vi "Drag-Drop Change.vi"(7 "Action":T1, 10 "Mouse Interaction Tag":string, 11 "UI Data In":refnum<class "Settings UI.lvclass">) -> (3 "UI Data Out":refnum<class "Settings UI.lvclass">)   [LabVIEW 2020, in "Output Sequencer.lvlib" / "Settings UI.lvclass"]
uses:
  Settings UI.lvclass
  Types/Settings UI Action.ctl
  Settings UI.lvclass/Settings UI.ctl
  Types/Drag-Drop State.ctl
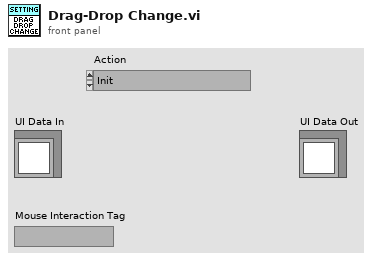
[diagram p1: front panel]
types:
  T1 = typedef "Output Sequencer.lvlib/Settings UI.lvclass/Settings UI Action.ctl" = enum16{"Init", "Timeout", "Tree Change", "Tree Mouse Down/Up", "Value Change", "Expand All", "Show Overview", "Collapse All", "Insert Above", "Insert Below", "Remove Step", "Move Up", "Move Down", "Drag Starting", "Drag Over", "Drop", "Drag Ended", "Import"}
  T2 = typedef "Output Sequencer.lvlib/Settings UI.lvclass/Drag-Drop State.ctl" = cluster{"Step Number":i32, "Current Index":i32, "Dropped?":bool, "Previous Open State":bool[]}
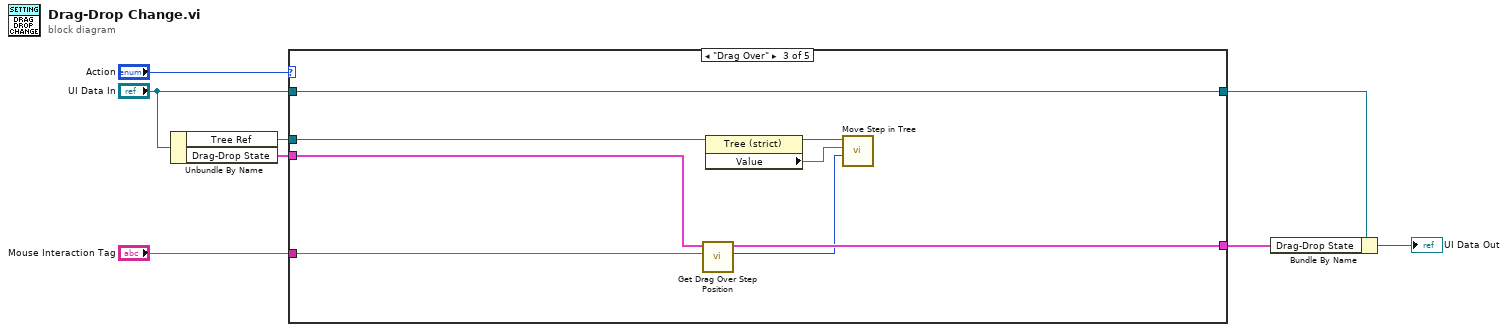
[diagram p0: block diagram]
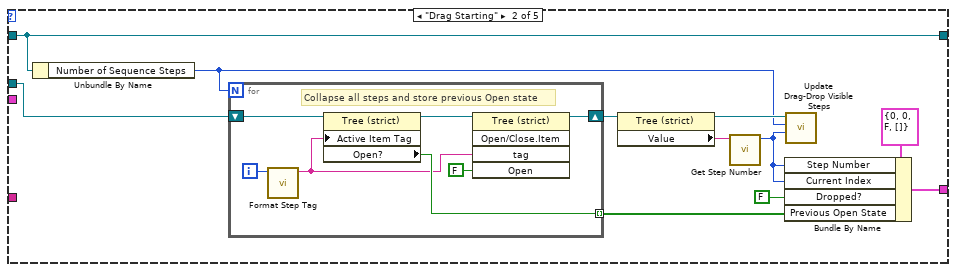
[diagram p3: hidden frame]
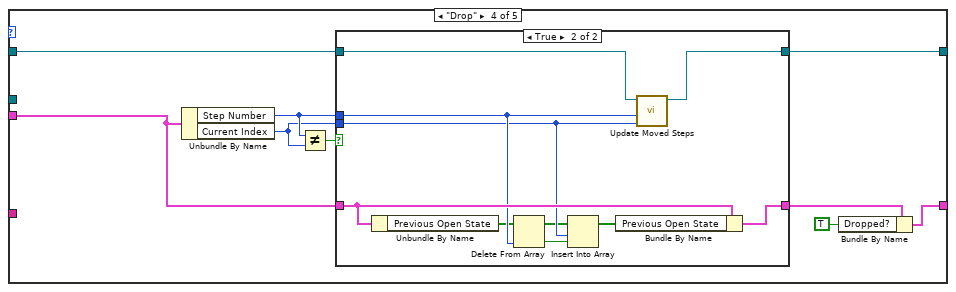
[diagram p4: hidden frame]
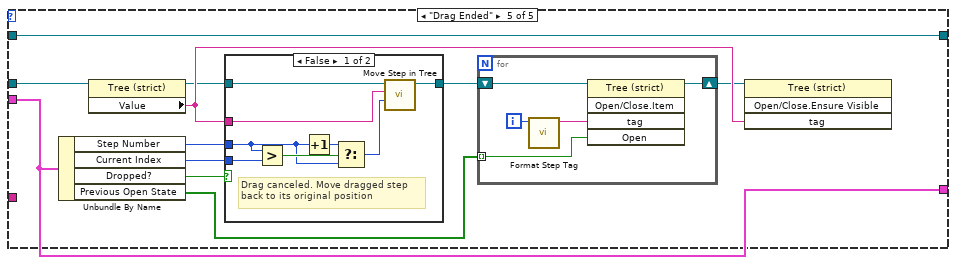
[diagram p6: hidden frame]
diagram:
  n1 = Unbundle By Name("UI Data In") -> ("Tree Ref"=w5:refnum<vi>, "Drag-Drop State"=w4:T2)
  n2 = case shown="\"Drag Over\"" "Action" {
    tunnel: w4 -> [w10 _ w35 w39 w67]
    tunnel: [w10 w19 w32 w37 w67] -> w1
    tunnel: "Mouse Interaction Tag" -> [_ _ w36 _ _]
    tunnel: "UI Data In" -> [w9 w18 w34 w44 w64]
    tunnel: [w9 w18 w34 w40 w64] -> w3
    tunnel: w5 -> [_ w11 w31 _ w58]
    frame Default {
    }
    frame "Drag Starting" {
      n3 = Unbundle By Name(w18) -> ("Number of Sequence Steps"=w13:i32)
      n4 = for {
        N: w13 -> [_]
        shift-right: [w27] -> w15
        shift-left: w11 -> [w26]
        tunnel: [w24] -> w17 mode=indexing
        i -> [w22]
        # "Collapse all steps and store previous Open state"
        n5 = call "Format Step Tag.vi"("Step Number"=w22) -> ("Tag"=w23:string)  [unwired: 10 in]
        n6 = property class="Tree (strict)"(reference=w26, "Active Item Tag"=w23) -> (reference out=w25:refnum<vi>, "Open?"=w24:bool)  [unwired: 1 in, 1 out]
        n7 = invoke class="Tree (strict)" method="Open/Close.Item"(reference=w25, "tag"=w23, "Open"=FALSE ("Open?")) -> (reference out=w27:refnum<vi>)  [unwired: 2 in, 4 out]
      }
      n8 = property class="Tree (strict)"(reference=w15) -> (reference out=w14:refnum<vi>, "Value"=w21:string)  [unwired: 1 in, 1 out]
      n9 = call "Get Step Number.vi"("Tree Tag"=w21) -> ("Step Number"=w12:i32)  [unwired: 8 in, 2 out]
      n10 = Bundle By Name(cluster=T2 {"Step Number"=0, "Current Index"=0, "Dropped?"=FALSE, "Previous Open State"=[]} ("Drag-Drop State in"), "Step Number"=w12, "Current Index"=w12, "Dropped?"=FALSE, "Previous Open State"=w17) -> (w19:T2)
      n11 = call "Update Drag-Drop Visible Steps.vi"("Step Number"=w12, "Number of Sequence Steps"=w13, "TreeControl in"=w14) -> ()  [unwired: 9 in]
    }
    frame "Drag Over" {
      n12 = call "Get Drag Over Step Position.vi"("Mouse Interaction Tag"=w36, "Drag-Drop State in"=w35) -> ("New Position"=w29:i32, "Drag-Drop State out"=w32:T2)  [unwired: 8 in]
      n13 = property class="Tree (strict)"(reference=w31) -> (reference out=w33:refnum<vi>, "Value"=w30:string)  [unwired: 1 in, 1 out]
      n14 = call "Move Step in Tree.vi"("New Position"=w29, "Step Tag"=w30, "TreeControl in"=w33) -> ()  [unwired: 8 in, 1 out]
    }
    frame "Drop" {
      n15 = Unbundle By Name(w39) -> ("Step Number"=w43:i32, "Current Index"=w42:i32)
      n16 = Not Equal?(x=w43, y=w42) -> (x != y?=w41:bool)
      n17 = case shown="True" w41 {
        tunnel: w44 -> [w47 w49]
        tunnel: w42 -> [_ w55]
        tunnel: w43 -> [_ w56]
        tunnel: [w47 w48] -> w40
        tunnel: w39 -> [w46 w57]
        tunnel: [w46 w54] -> w38
        frame False {
        }
        frame True {
          n18 = Unbundle By Name(w57) -> ("Previous Open State"=w53:bool[])
          n19 = Delete From Array(array=w53, index=w56) -> (deleted portion=w51:bool, array with subset deleted=w52:bool[])  [unwired: 1 in]
          n20 = Insert Into Array(array=w52, index=w55, new element=w51) -> (w50:bool[])
          n21 = Bundle By Name(cluster=w57, "Previous Open State"=w50) -> (w54:T2)
          n22 = call "Update Moved Steps.vi"("New Step Number"=w55, "Previous Step Number"=w56, "UI Data In"=w49) -> ("UI Data Out"=w48:refnum<class "Settings UI.lvclass">)  [unwired: 8 in]
        }
      }
      n23 = Bundle By Name(cluster=w38, "Dropped?"=TRUE) -> (w37:T2)
    }
    frame "Drag Ended" {
      n24 = Unbundle By Name(w67) -> ("Step Number"=w65:i32, "Current Index"=w66:i32, "Dropped?"=w60:bool, "Previous Open State"=w59:bool[])
      n25 = property class="Tree (strict)"(reference=w58) -> (reference out=w61:refnum<vi>, "Value"=w68:string)  [unwired: 1 in, 1 out]
      n26 = case shown="False" w60 {
        tunnel: w61 -> [w75 w82]
        tunnel: [w74 w82] -> w62
        tunnel: w68 -> [w77 _]
        tunnel: w66 -> [w79 _]
        tunnel: w65 -> [w78 _]
        frame False {
          # "Drag canceled. Move dragged step\nback to its original position"
          n27 = Greater?(x=w78, y=w79) -> (0:w81:bool)
          n28 = Increment(x=w78) -> (x+1=w80:i32)
          n29 = Select(t=w80, s=w81, f=w78) -> (s? t:f=w76:i32)
          n30 = call "Move Step in Tree.vi"("New Position"=w76, "Step Tag"=w77, "TreeControl in"=w75) -> ("TreeControl out"=w74:refnum<vi>)  [unwired: 8 in]
        }
        frame True {
        }
      }
      n31 = for {
        shift-right: [w73] -> w63
        shift-left: w62 -> [w72]
        tunnel: w59 -> [w71] mode=indexing
        i -> [w70]
        n32 = call "Format Step Tag.vi"("Step Number"=w70) -> ("Tag"=w69:string)  [unwired: 10 in]
        n33 = invoke class="Tree (strict)" method="Open/Close.Item"(reference=w72, "tag"=w69, "Open"=w71) -> (reference out=w73:refnum<vi>)  [unwired: 2 in, 4 out]
      }
      n34 = invoke class="Tree (strict)" method="Open/Close.Ensure Visible"(reference=w63, "tag"=w68) -> ()  [unwired: 2 in, 4 out]
    }
  }
  n35 = Bundle By Name(cluster=w3, "Drag-Drop State"=w1) -> (→"UI Data Out":refnum<class "Settings UI.lvclass">)
